vi "MustLock.vi"(1 "SurfaceFlags":T1 items=["SDL_SURFACE_PREALLOCATED"=1, "SDL_SURFACE_LOCK_NEEDED"=2, "SDL_SURFACE_LOCKED"=4, "SDL_SURFACE_SIMD_ALIGNED"=8]) -> (0 "Must Lock?":bool)   [LabVIEW 2024, in "SDL3.lvlib" / "Surface.lvlib"]
doc: "<B>Summary</B>\nEvaluates to true if the surface needs to be locked before access.\n\n<B>LV Implementation</B>\nTakes SurfaceFlags instead of Surface to reduce memory dereferencing."
uses:
  Surface.lvlib
  SurfaceFlags--ring.ctl
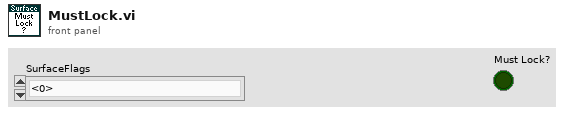
[diagram p1: front panel]
types:
  T1 = typedef "SDL3.lvlib/Surface.lvlib/SurfaceFlags--ring.ctl" = u32
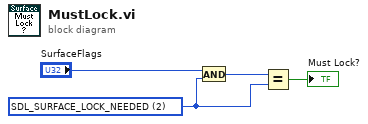
[diagram p0: block diagram]
diagram:
  w2 = T1 2 items=["SDL_SURFACE_PREALLOCATED"=1, "SDL_SURFACE_LOCK_NEEDED"=2, "SDL_SURFACE_LOCKED"=4, "SDL_SURFACE_SIMD_ALIGNED"=8] ("SurfaceFlags")
  n1 = And(x="SurfaceFlags", y=w2) -> (x .and. y?=w3:T1)
  n2 = Equal?(x=w3, y=w2) -> (x = y?=→"Must Lock?":bool)
